vi "Keithley 2400 Test.vi"() -> ()   [LabVIEW 2011]
uses:
  <instrlib>/keithley_24xx/Keithley 24XX/Public/Data/Read (Single Point).vi
  <instrlib>/keithley_24xx/Keithley 24XX/Keithley 24XX.lvlib
panel:
  in  "STOP":bool
  in  "Keithley 2400 Address 2":refnum<visa-resource-name>="GPIB0::26::INSTR"
  in  "Source Mode":enum16{"Voltage", "Current"}(ring)
  in  "Top Electrode Level (V or A)":dbl
  in  "Turn off Keithley":bool
  in  "Turn on Keithley":bool
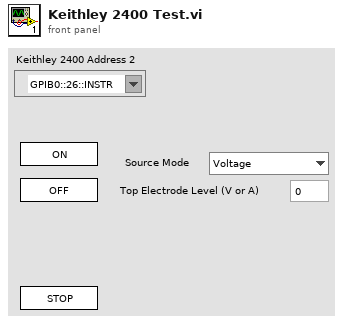
[diagram p1: front panel]
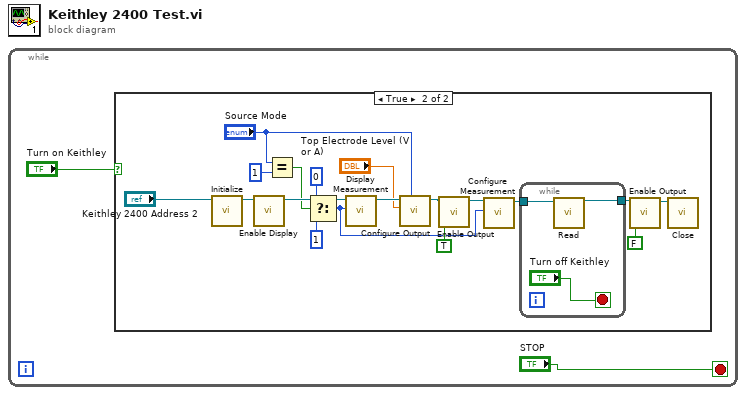
[diagram p0: block diagram]
diagram:
  n1 = while {
    stop <- "STOP" stop-if-true
    n2 = case shown="True" "Turn on Keithley" {
      frame False {
      }
      frame True {
        n3 = call <instrlib>:"Initialize.vi"("VISA resource name"="Keithley 2400 Address 2") -> ("VISA resource name out"=w17:refnum<visa-resource-name>)  [unwired: 4 in, 6 out]
        n4 = call <instrlib>:"Enable Display.vi"("VISA resource name"=w17) -> ("VISA resource name out"=w18:refnum<visa-resource-name>)  [unwired: 2 in, 8 out]
        n5 = Equal?(x="Source Mode", y=i16 1) -> (x = y?=w11:bool)
        n6 = Select(t=0, s=w11, f=1) -> (s? t:f=w7:i32)
        n7 = call <instrlib>:"Display Measurement.vi"("Displayed Measurement (0: Voltage)"=w7, "VISA resource name"=w18) -> ("VISA resource name out"=w19:refnum<visa-resource-name>)  [unwired: 1 in, 8 out]
        n8 = call <instrlib>:"Configure Output.vi"("Source Mode  (0: Voltage)"="Source Mode", "Output Level (0)"="Top Electrode Level (V or A)", "VISA resource name"=w19) -> ("VISA resource name out"=w9:refnum<visa-resource-name>)  [unwired: 3 in, 5 out]
        n9 = call <instrlib>:"Enable Output.vi"("Enable Output (T: Enable)"=TRUE ("reset device (true)"), "VISA resource name"=w9) -> ("VISA resource name out"=w8:refnum<visa-resource-name>)  [unwired: 1 in, 8 out]
        n10 = call <instrlib>:"Configure Measurement.vi"("Function (0: Volts)"=w7, "VISA resource name"=w8) -> ("VISA resource name out"=w6:refnum<visa-resource-name>)  [unwired: 3 in, 6 out]
        n11 = while {
          tunnel: w6 -> [w23]
          tunnel: [w22] -> w3
          stop <- "Turn off Keithley" stop-if-true
          n12 = call-poly <instrlib>:"Read.vi"("VISA resource name"=w23) -> ("VISA resource name out"=w22:refnum<visa-resource-name>)  [unwired: 8 in, 6 out]
        }
        n13 = call <instrlib>:"Enable Output.vi"("Enable Output (T: Enable)"=FALSE ("reset device (true)"), "VISA resource name"=w3) -> ("VISA resource name out"=w5:refnum<visa-resource-name>)  [unwired: 1 in, 8 out]
        n14 = call <instrlib>:"Close.vi"("VISA resource name"=w5) -> ()  [unwired: 10 in, 1 out]
      }
    }
  }
